vi "Read Read Only.vi"(8 "error in (no error)":errorcluster, 11 "Const_CPLX_SGL in":refnum<class "Const_CPLX_SGL.lvclass">) -> (0 "error out":errorcluster, 2 "Read Only":bool, 3 "Const_CPLX_SGL out":refnum<class "Const_CPLX_SGL.lvclass">)   [LabVIEW 2021, in "Const_CPLX_SGL.lvclass"]
uses:
  Const_CPLX_SGL.lvclass
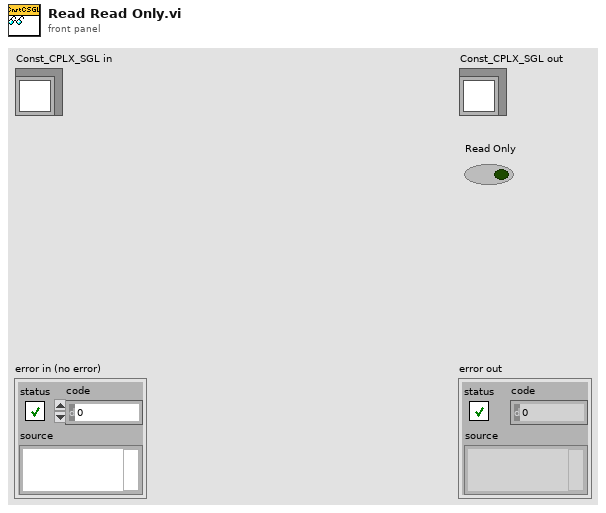
[diagram p1: front panel]
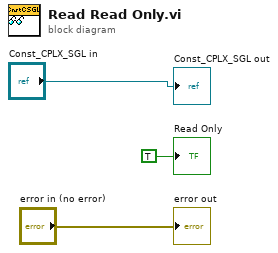
[diagram p0: block diagram]
diagram:
  "error out" <- "error in (no error)"
  "Const_CPLX_SGL out" <- "Const_CPLX_SGL in"
  "Read Only" <- TRUE ("Read Only")
